vi "ReadDBL Array.vi"(6 "length":u16, 8 "error in (no error)":errorcluster, 10 "Start address":string, 11 "MelsecTCP in":refnum<class "Abs Controler.lvclass">) -> (0 "error out":errorcluster, 2 "Data":dbl[](array[numeric]), 3 "MelsecTCP out":refnum<class "Abs Controler.lvclass">)   [LabVIEW 2020, in "HslCommunication.lvlib" / "Abs Controler.lvclass"]
uses:
  Abs Controler.lvclass
  E:/Git/Libraries/develop/HslCommunication/_Dependenciecs/HslCommunication.dll
  _Dependenciecs/HslCommunication.dll
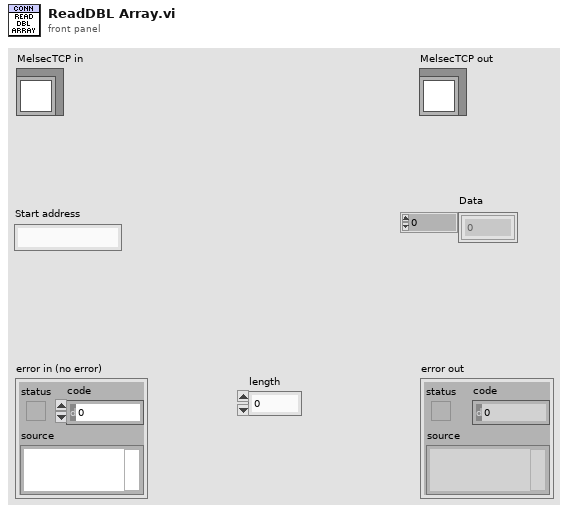
[diagram p1: front panel]
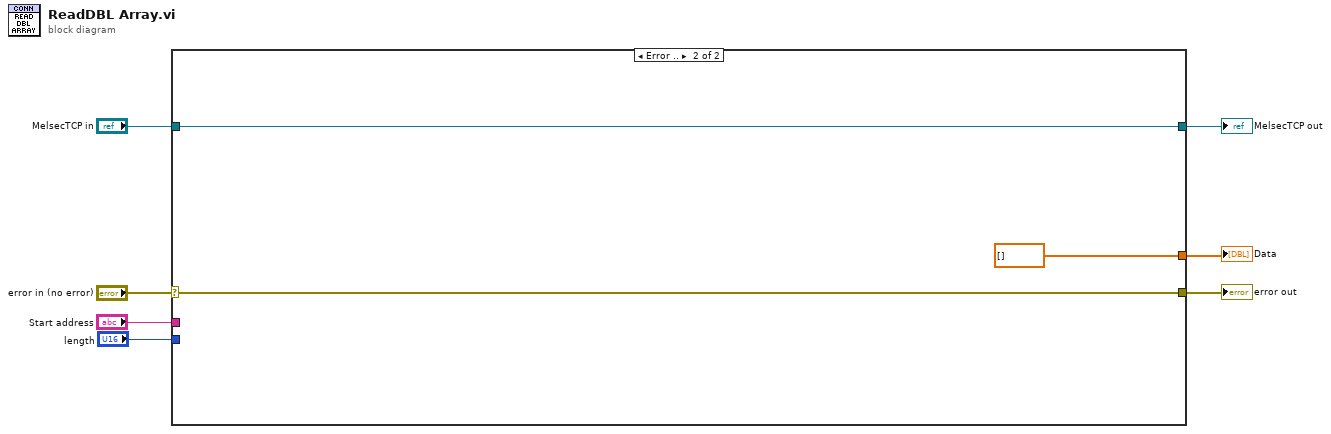
[diagram p0: block diagram]
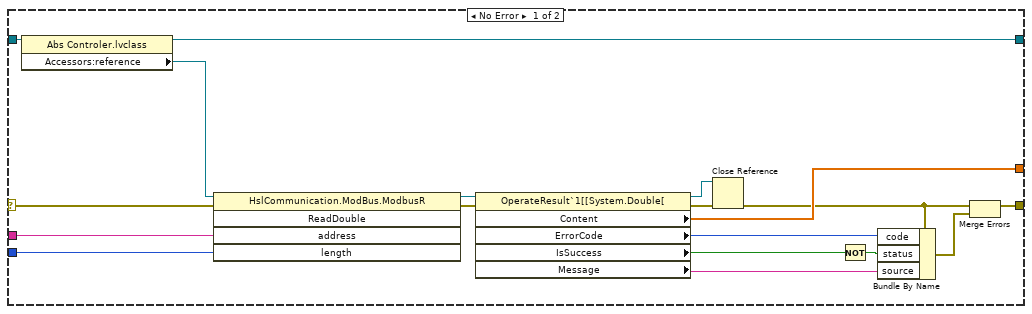
[diagram p2: hidden frame]
diagram:
  n1 = case shown="Error .." "error in (no error)" {
    selector: "error in (no error)" -> [w14 w28]
    tunnel: "MelsecTCP in" -> [w25 w27]
    tunnel: [w16 w27] -> w3
    tunnel: "Start address" -> [w15 _]
    tunnel: [w22 w28] -> w4
    tunnel: [w23 dbl[] [] ("Content")] -> w2
    tunnel: "length" -> [w8 _]
    frame No Error {
      n2 = property class="Abs Controler.lvclass"(reference=w25) -> (reference out=w16:refnum<class "Abs Controler.lvclass">, "Accessors:reference"=w24:refnum<k24>)  [unwired: 1 in, 1 out]
      n3 = invoke class="HslCommunication.ModBus.ModbusR" method="ReadDouble"(reference=w24, error in=w14, "address"=w15, "length"=w8) -> (error out=w12:errorcluster, "ReadDouble"=w10:refnum<k24>)  [unwired: 1 in, 3 out]
      n4 = property class="OperateResult`1[[System.Double["(reference=w10, error in=w12) -> (reference out=w9:refnum<k24>, error out=w11:errorcluster, "Content"=w23:dbl[], "ErrorCode"=w21:i32, "IsSuccess"=w20:bool, "Message"=w19:string)
      n5 = Close Reference(reference=w9, error in (no error)=w11) -> (error out=w18:errorcluster)
      n6 = Not(x=w20) -> (.not. x?=w13:bool)
      n7 = Bundle By Name(cluster=w18, "code"=w21, "status"=w13, "source"=w19) -> (w17:errorcluster)
      n8 = Merge Errors(w18, w17) -> (w22:errorcluster)
    }
    frame Error {
    }
  }
  "error out" <- w4
  "MelsecTCP out" <- w3
  "Data" <- w2
